vi "Close.vi"(8 "error in (no error)":errorcluster) -> (0 "error out":errorcluster)   [LabVIEW 2019, in "输出轴伺服.lvlib"]
uses:
  Servo_global.vi
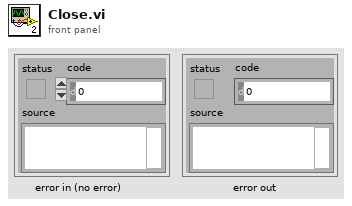
[diagram p1: front panel]
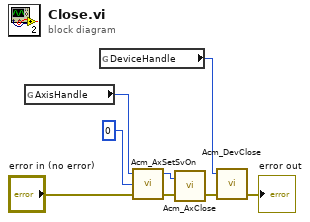
[diagram p0: block diagram]
diagram:
  n1 = global read "Servo_global.vi" "AxisHandle"() -> (w3:u32)
  n2 = global read "Servo_global.vi" "DeviceHandle"() -> (w6:u32)
  n3 = call <userlib>:"Acm_AxSetSvOn.vi"("error in (no error)"="error in (no error)", "OnOff"=u32 0, "AxisHandle"=w3) -> ("error out"=w1:errorcluster, "AxisHandle"=w2:u32)  [unwired: 1 out]
  n4 = call <userlib>:"Acm_AxClose.vi"("error in (no error)"=w1, "AxisHandle"=w2) -> ("error out"=w8:errorcluster)  [unwired: 1 out]
  n5 = call <userlib>:"Acm_DevClose.vi"("error in (no error)"=w8, "DeviceHandle"=w6) -> ("error out"=→"error out":errorcluster)  [unwired: 2 in, 1 out]
